vi "FGV_PROXY_DIAGNOSTICS_single_message_display.vi"(4 "front_panel_reference":refnum<vi>, 6 "SQL_listbox_reference":refnum<vi>, 7 "options":T2, 8 "error_in":errorcluster, 9 "station":T1, 11 "input":variant) -> (0 "error_out":errorcluster)   [LabVIEW 2020]
uses:
  FGV_PROXY_DIAGNOSTICS_single_message_display.ctl
  STATION/station.ctl
  _misc/AULocalize/SubVIs/Get Localized Phrase Compact Interface 1D.vi
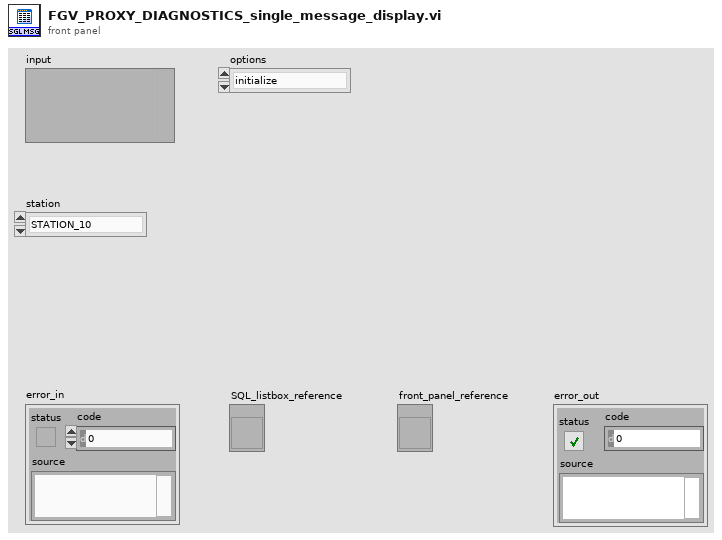
[diagram p1: front panel]
types:
  T1 = typedef "station.ctl" = enum16{"STATION_10", "STATION_20", "STATION_30", "STATION_40", "STATION_50", "STATION_60", "STATION_70", "STATION_80", "STATION_90", "STATION_100", "STATION_110", "STATION_120", "STATION_165", "MAIN"}
  T2 = typedef "FGV_PROXY_DIAGNOSTICS_single_message_display.ctl" = enum16{"initialize", "display_message"}
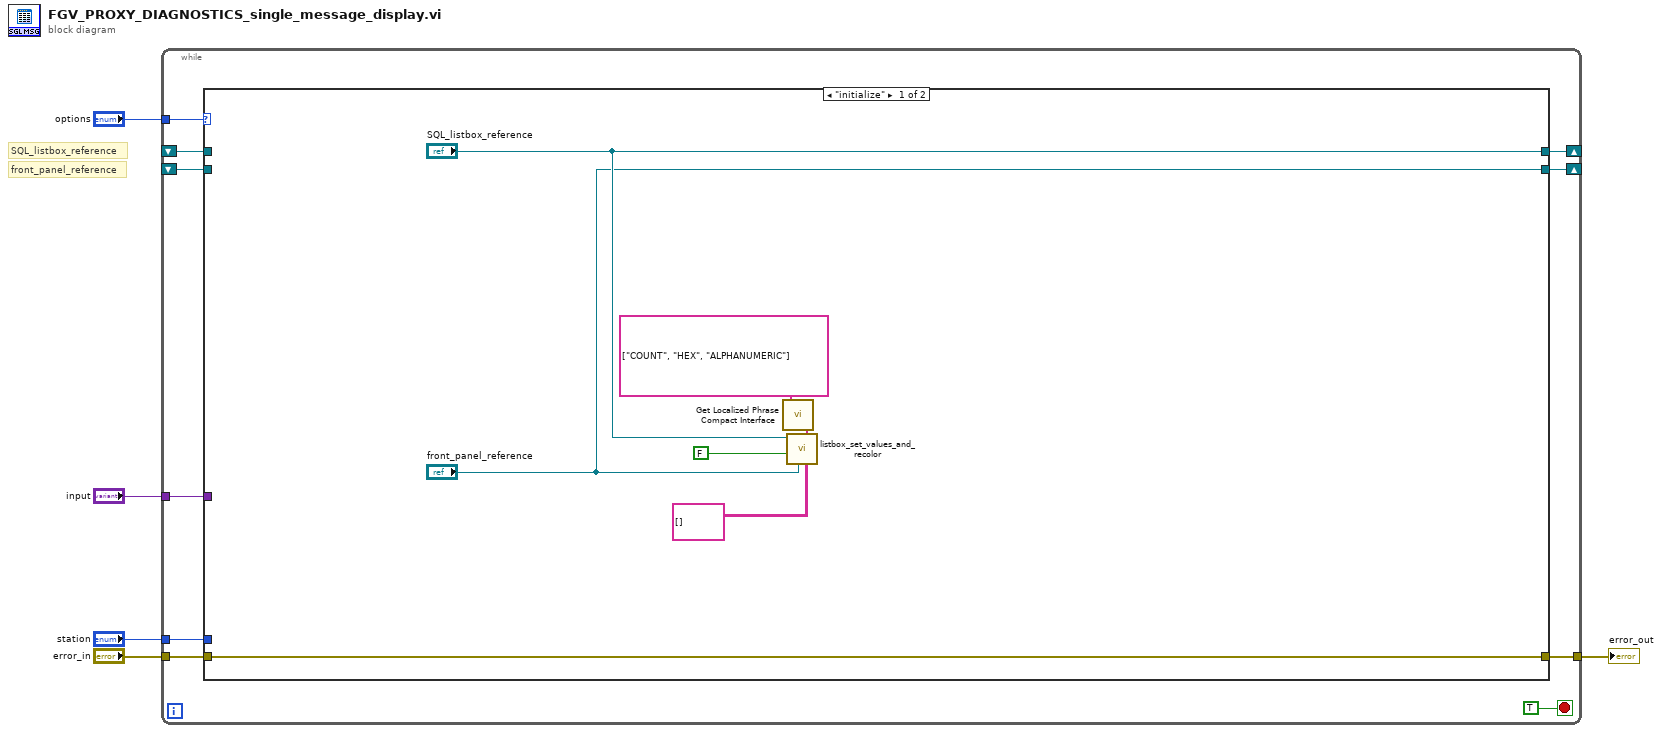
[diagram p0: block diagram]
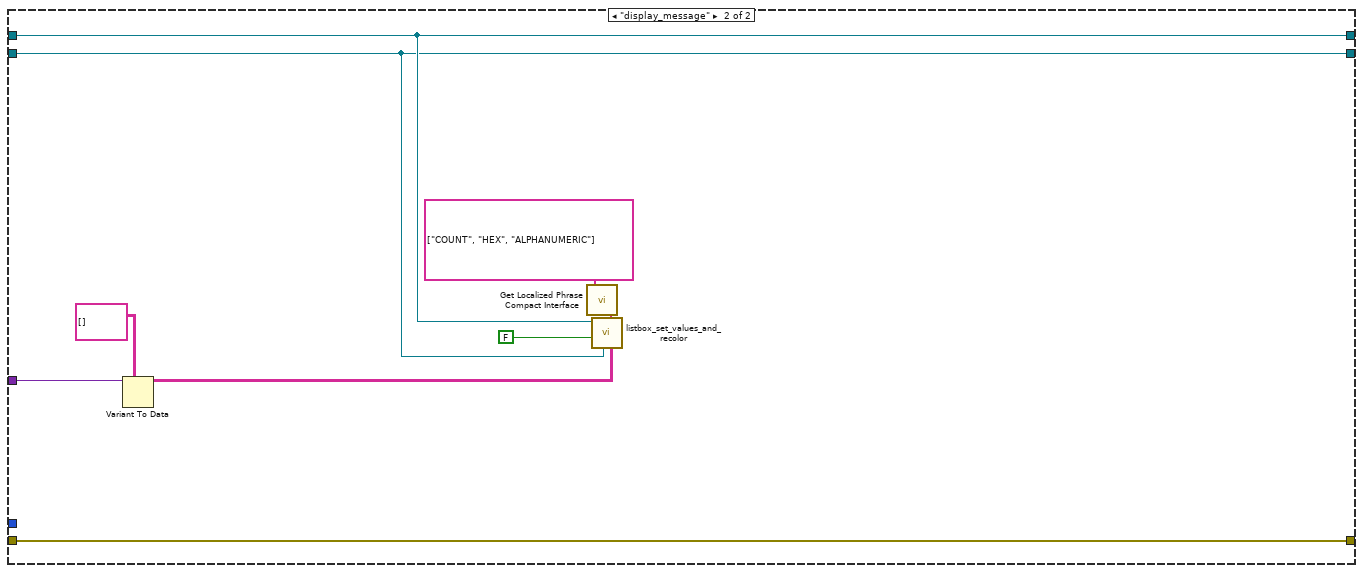
[diagram p2: hidden frame]
diagram:
  # "front_panel_reference"
  # "SQL_listbox_reference"
  n1 = while {
    tunnel: "options" -> [w14]
    tunnel: [w13] -> w5
    tunnel: "error_in" -> [w12]
    shift-right: [w11] -> _
    shift-left: _ -> [w10]
    tunnel: "input" -> [w9]
    shift-right: [w8] -> _
    shift-left: _ -> [w7]
    tunnel: "station" -> [w6]
    stop <- TRUE stop-if-true
    n2 = case shown="\"initialize\"" w14 {
      tunnel: [w22 w31] -> w13
      tunnel: w12 -> [w22 w31]
      tunnel: ["SQL_listbox_reference" w28] -> w11
      tunnel: w10 -> [_ w28]
      tunnel: w9 -> [_ w26]
      tunnel: ["front_panel_reference" w27] -> w8
      tunnel: w7 -> [_ w27]
      tunnel: w6 -> [_ _]
      frame "initialize" {
        n3 = call-poly "Get Localized Phrase Compact Interface.vi"("Key"=string[] ["COUNT", "HEX", "ALPHANUMERIC"] ("column_names")) -> ("Translated Phrase"=w16:string[])
        n4 = call "listbox_set_values_and_recolor.vi"("item_names"=string[][] [], "front_panel_reference"="front_panel_reference", "column_names"=w16, "Autosize? (T)"=FALSE, "multicolumn_listbox_reference_in"="SQL_listbox_reference") -> ()  [unwired: 5 in, 2 out]
      }
      frame "display_message" {
        n5 = Variant To Data(type=string[][] [] ("item_names"), Variant=w26) -> (data=w24:string[][])  [unwired: 1 in, 1 out]
        n6 = call-poly "Get Localized Phrase Compact Interface.vi"("Key"=string[] ["COUNT", "HEX", "ALPHANUMERIC"] ("column_names")) -> ("Translated Phrase"=w23:string[])
        n7 = call "listbox_set_values_and_recolor.vi"("item_names"=w24, "front_panel_reference"=w27, "column_names"=w23, "Autosize? (T)"=FALSE, "multicolumn_listbox_reference_in"=w28) -> ()  [unwired: 5 in, 2 out]
      }
    }
  }
  "error_out" <- w5
